vi "Add Cast If Needed.vi"(7 "JSON Type String":string, 9 "Literal Value Ctl Ref":T1, 10 "Build Array Term Ref":refnum<vi>, 11 "Diagram":T2) -> (3 "PolymorphicSubVI out":refnum<vi>)   [LabVIEW 2015, in "Build JSON Array.xnode"]
doc: "Adds a typecast to the JSON object\n\nDO NOT USE"
uses:
  Build JSON Array.xnode
  <vilib>/XNodeSupport/XNodeTopLevelDiagramRef.ctl
  <vilib>/XNodeSupport/XNodeTermRef.ctl
  <vilib>/Utility/miscctls.llb/LVPointTypeDef.ctl
  JSON Helper/New JSON.vi
  JSON Helper/JSON Helper.lvclass
  <vilib>/XNodeSupport/NI_XNodeSupport.lvlib
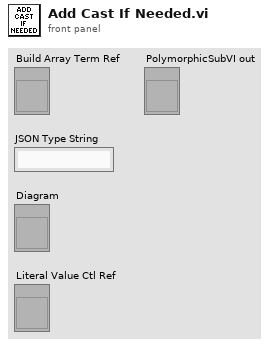
[diagram p1: front panel]
types:
  T1 = typedef "NI_XNodeSupport.lvlib/XNodeTermRef.ctl" = refnum<vi>
  T2 = typedef "NI_XNodeSupport.lvlib/XNodeTopLevelDiagramRef.ctl" = refnum<vi>
  T3 = typedef "LVPointTypeDef.ctl" = cluster{"Horizontal":i16, "Vertical":i16}
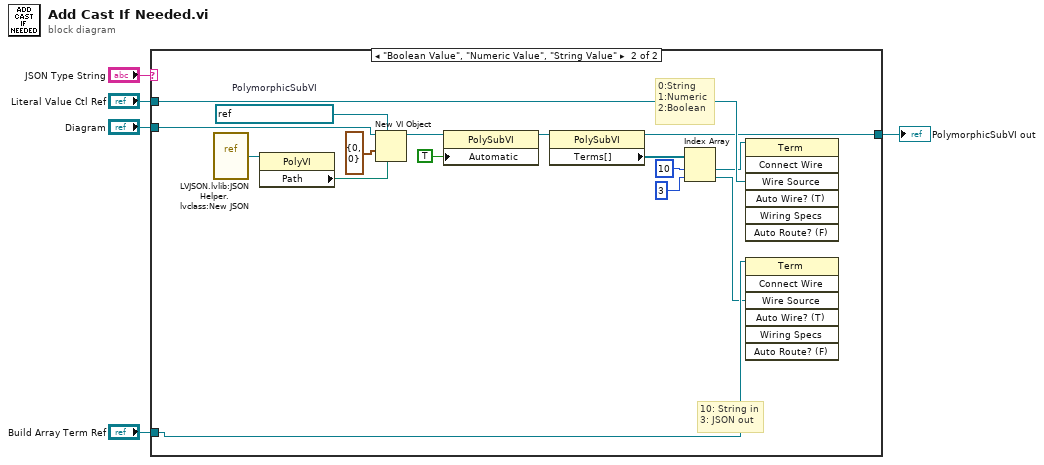
[diagram p0: block diagram]
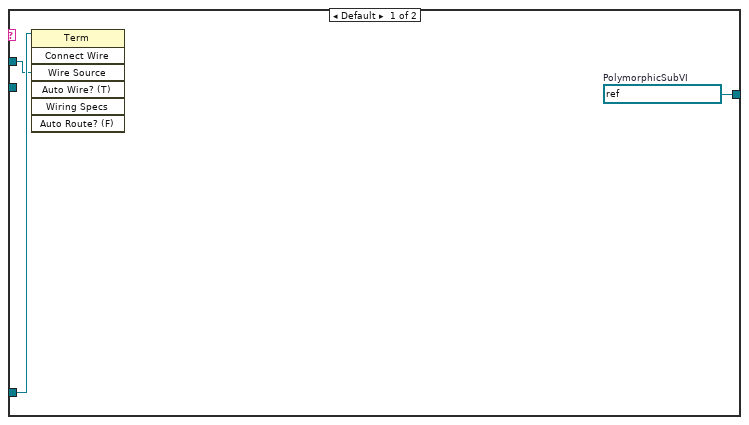
[diagram p2: hidden frame]
diagram:
  n1 = case shown="\"Boolean Value\", \"Numeric Value\", \"String Value\"" "JSON Type String" {
    tunnel: "Build Array Term Ref" -> [w8 w12]
    tunnel: "Literal Value Ctl Ref" -> [w7 w24]
    tunnel: "Diagram" -> [_ w19]
    tunnel: [w6 w9] -> w5
    frame Default {
      w6 = refnum<vi> refnum  # PolymorphicSubVI
      n2 = invoke class="Term" method="Connect Wire"(reference=w8, "Wire Source"=w7) -> ()  [unwired: 5 in, 7 out]
    }
    frame "Boolean Value", "Numeric Value", "String Value" {
      w21 = refnum<vi> refnum  # PolymorphicSubVI
      # "10: String in\n3: JSON out"
      # "0:String\n1:Numeric\n2:Boolean"
      n3 = vi-ref "LVJSON.lvlib:JSON Helper.lvclass:New JSON.vi"() -> (w18:refnum<vi>)
      n4 = property class="PolyVI"(reference=w18) -> ("Path"=w22:path)  [unwired: 1 in, 2 out]
      n5 = New VI Object(vi object class=w21, owner refnum=w19, position/next to=T3 {"Horizontal"=0, "Vertical"=0} ("location"), 6:w22) -> (object refnum=w23:refnum<vi>)  [unwired: 4 in, 1 out]
      n6 = property class="PolySubVI"(reference=w23, "Automatic"=TRUE) -> (reference out=w17:refnum<vi>)  [unwired: 1 in, 1 out]
      n7 = property class="PolySubVI"(reference=w17) -> (reference out=w9:refnum<vi>, "Terms[]"=w16:refnum<vi>[])  [unwired: 1 in, 1 out]
      n8 = Index Array(array=w16, index #1=10 ("index"), index #2=3 ("index")) -> (element #1=w13:refnum<vi>, element #2=w11:refnum<vi>)
      n9 = invoke class="Term" method="Connect Wire"(reference=w13, "Wire Source"=w24) -> ()  [unwired: 5 in, 7 out]
      n10 = invoke class="Term" method="Connect Wire"(reference=w12, "Wire Source"=w11) -> ()  [unwired: 5 in, 7 out]
    }
  }
  "PolymorphicSubVI out" <- w5
